vi "FormCalibra9.vi"() -> ()   [LabVIEW 2014]
uses:
  testMachine.ctl
  mainMachine.ctl
  <vilib>/Analysis/baseanly.llb/Mean (DBL).vi
  <vilib>/express/express shared/transition.llb/Dynamic To Waveform Array.vi
  <vilib>/express/express signal manip/GetorSetDDTAttributes/Set DDT Attributes/SetT0.vi
  <vilib>/express/express shared/transition.llb/Waveform Array To Dynamic.vi
  <vilib>/measure/mamon.llb/Trigger Detection for 1 Channel.vi
  <vilib>/express/express signal manip/GetorSetDDTAttributes/Set DDT Attributes/Set DDT Properties.xnode
  <vilib>/Analysis/NI_AALBase.lvlib
  <resource>/objmgr/daqmx.rc
  <vilib>/measure/NI_MAPro.lvlib
panel:
  out "editDistance":dbl caption="Distancia (m)" format="%#_4f"
  in  "Lower level":dbl
  in  "hysteresis":dbl format="%.2p"
  in  "level":dbl format="%.2p"
  out "rpm":bool
  out "deviceName":tag
  out "editTotalWaitLimit":u8
  out "editCountWaitLimit":u8
  out "ledWaitState":bool caption="Wait State"
  out "sliderWaitUpperTime":u8(slide) max=50 scale=0.0..100.0
  out "slideWaitLowerTime":u8(slide) max=30 scale=0.0..100.0
  out "slideWaitTime":u8(slide) scale=0.0..100.0
  out "labelTestTime":string caption="Tempo total de ensaio"
  in  "buttonAcquisition":bool
  in  "editSetWaitTime":u8 caption="Tempo entre ciclos (s)" step=1 format="%0d"
  in  "stop":bool
  out "error out":errorcluster
  out "ledAcquireState":bool caption="Acquire State"
  out "editTotalLowerLimit":u8
  out "editCountLowerLimit":u8
  out "editTotalUpperLimit":u8
  out "editCountUpperLimit":u8
  out "ledEnsaio 3":bool
  out "ledBrakeState":bool caption="Brake State"
  out "ledExitState":bool caption="Exit State"
  out "ledMotorState":bool caption="Motor State"
  out "ledInit2State":bool caption="Init State"
  out "ledBlockState":bool caption="Block State"
  out "ledRunningState":bool caption="Running State"
  out "ledReadyState":bool caption="Ready State"
  out "ledInitState":bool caption="Init State"
  out "mainMachine":T1
  out "testMachine":T2=enum."finish"
  in  "editSetPathToFile":path
  in  "buttonStop":bool
  in  "buttonStart":bool
  out "graphForce":dynamicdata(graph)
  in  "editOffsetForce":dbl caption="Tara" min=0.0 max=100.0 step=0.1
  in  "editSetForce":dbl caption="Fator de conversão"
  out "editForce":dbl caption="Força (Kgf)" format="%#_4f"
  out "graphSpeed":dynamicdata(graph)
  in  "editSetSpeed":dbl caption="Fator de conversão"
  out "editSpeed":dbl caption="Velocidade (km/h)" format="%#_4f"
  out "editEngineSpeed":dbl caption="Rotação (RPM)" format="%#_4f"
  in  "buttonMotor":bool
  in  "buttonBrake":bool
  in  "editSetWaitLowerTime":u8 caption="Tempo de espera (s)"
  in  "editSetWaitUpperTime":u8=3 caption="Tempo de espera (s)"
  in  "editSetNumberOfCycles":u16 caption="Número de ciclos" max=999 step=1 format="%0d"
  in  "editSetLowerLimit":u32 caption="Limite inferior (km/h)"
  in  "editSetUpperLimit":u32 caption="Limite superior (km/h)"
  out "editTempB":dbl caption="Temperatura B (ºC)"
  out "editTempA":dbl caption="Temperatura A (ºC)"
  in  "editSetTempRef":dbl caption="Offset referência" step=0.01 format="%#_2f"
  out "editTempRef":dbl caption="Referência (ºC)"
  out "ledMotor":bool
  out "ledBrake":bool
  out "ledEnsaio":bool
  out "labelTotalCycle":string
  out "labelCurrentCycle":string
  out "labelSystemTitle":string
  in  "editCurrCycleCtr":u32
  in  "velocidade 2":u32
  out "velocidade":u32
  # "Bancada de Frenagem - Ensaio"
  # "Ensaio"
  # "Temperatura"
  # "Rotação"
  # "Célula de Carga"
  # "Configurações do ensaio"
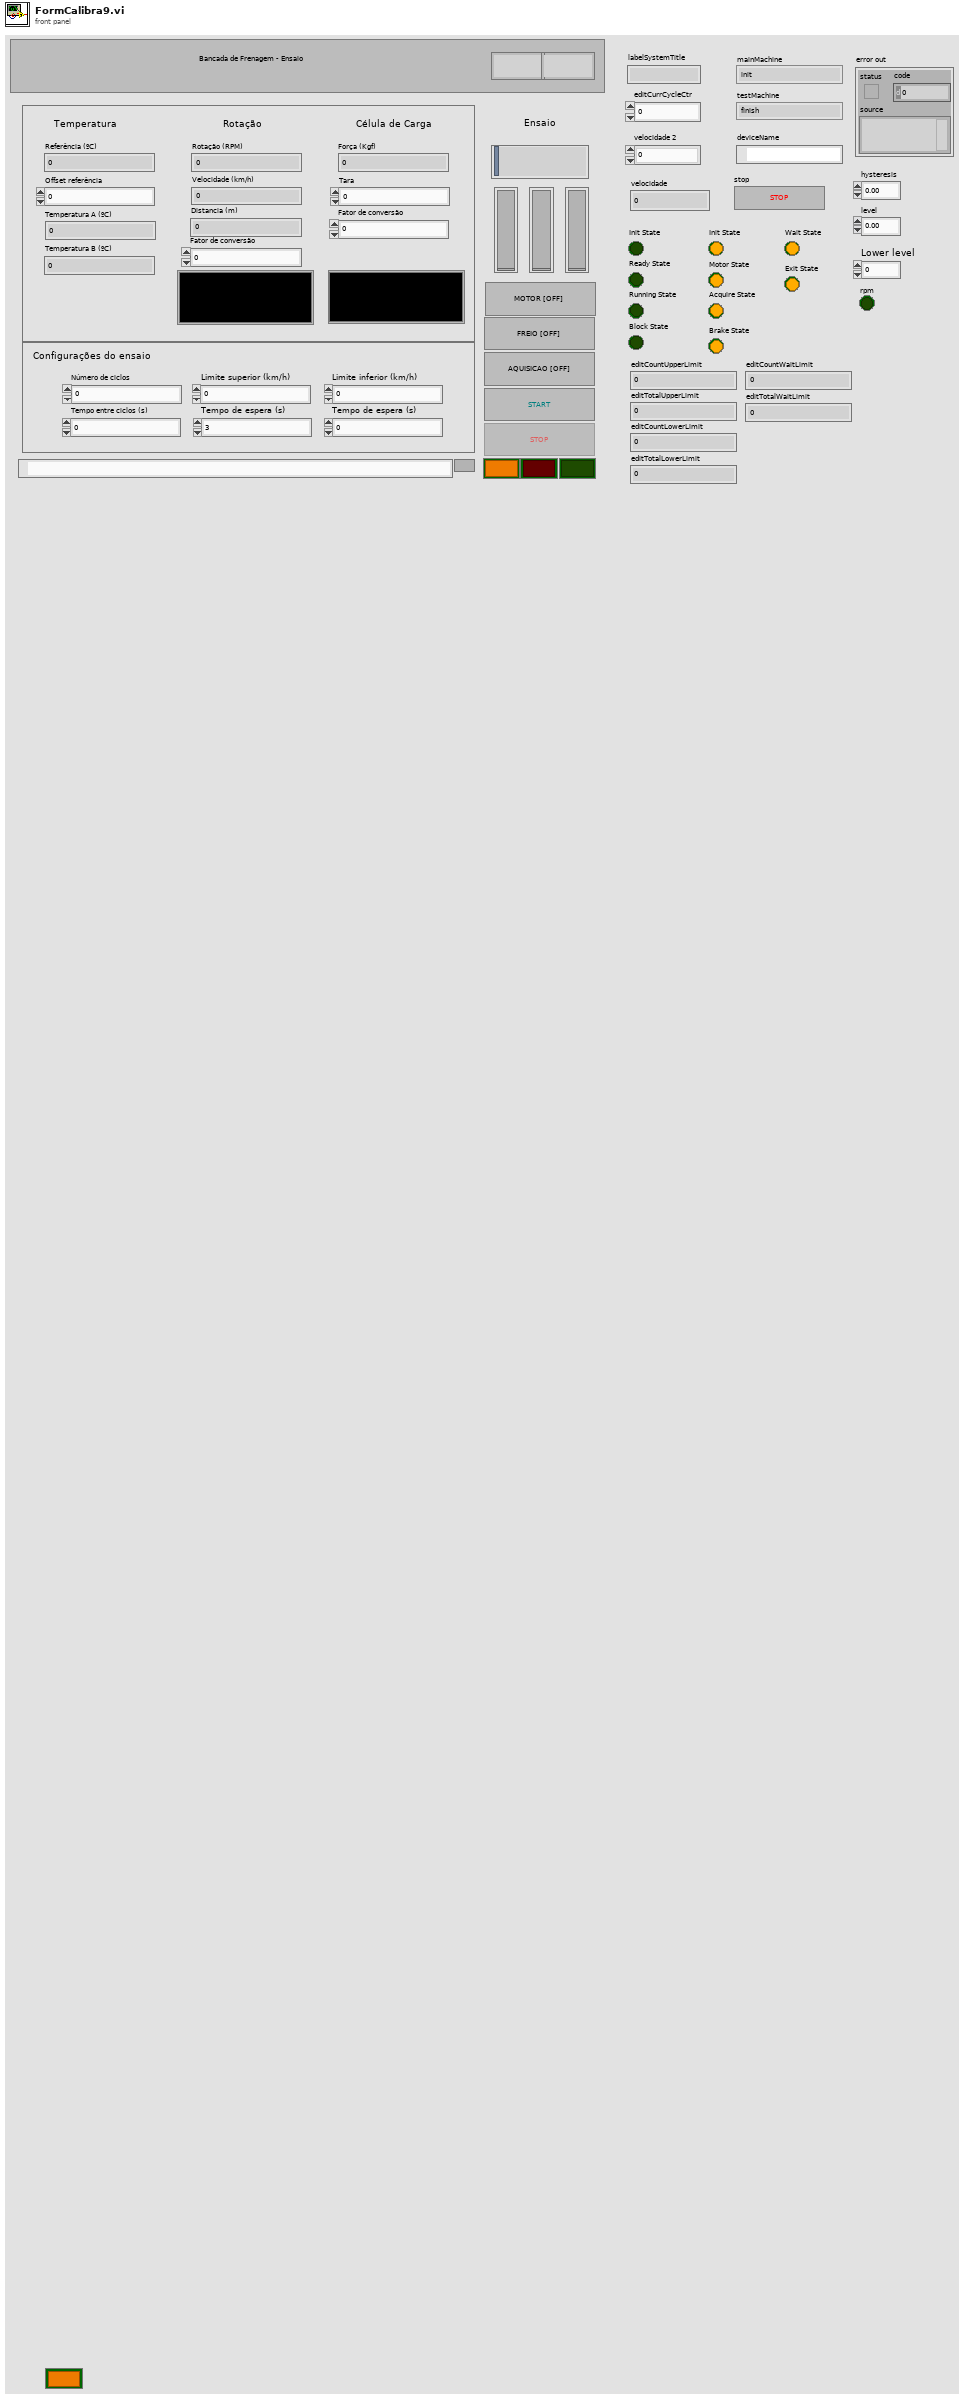
[diagram p1: front panel]
types:
  T1 = typedef "mainMachine.ctl" = enum16{"init", "ready", "running", "blocked", "finish"}
  T2 = typedef "testMachine.ctl" = enum16{"init", "motor", "motor acquire", "brake", "brake acquire", "wait ", "finish", "exit"}
  T3 = enum8{"Enabled", "Disabled", "Disabled and Grayed Out"}
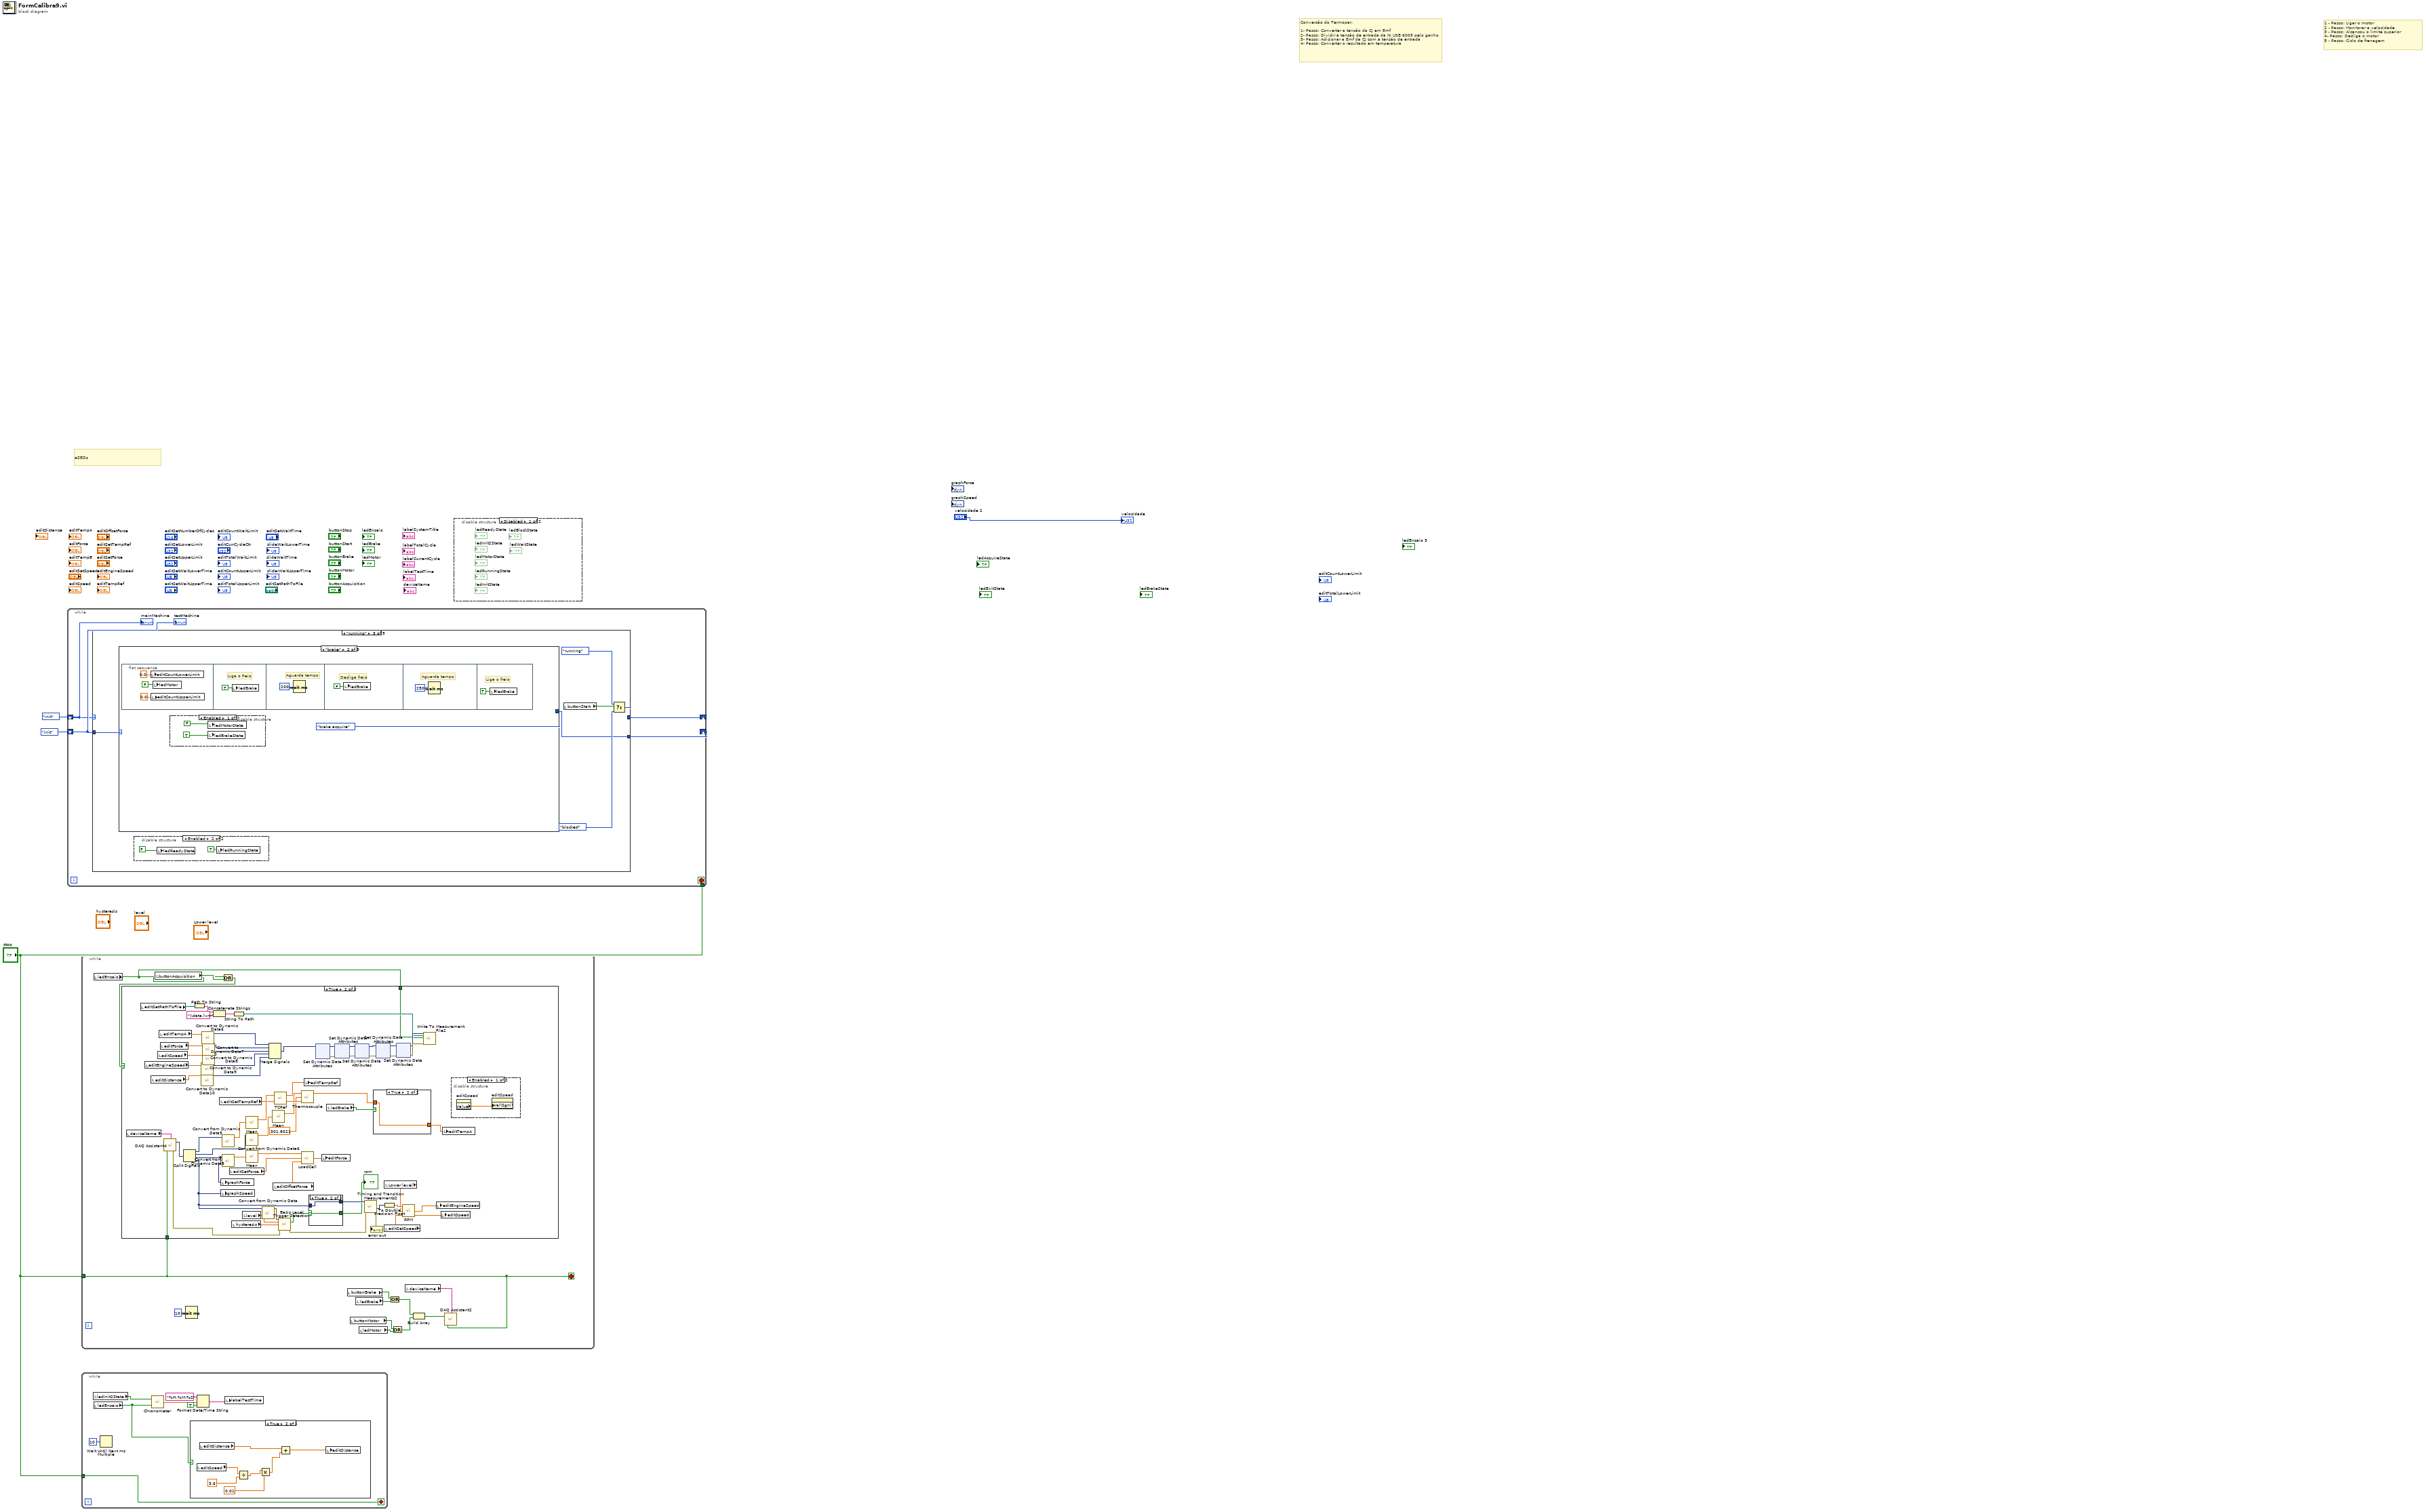
[diagram p0: block diagram]
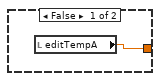
[diagram p5: hidden frame]
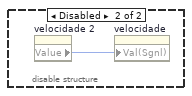
[diagram p7: hidden frame]
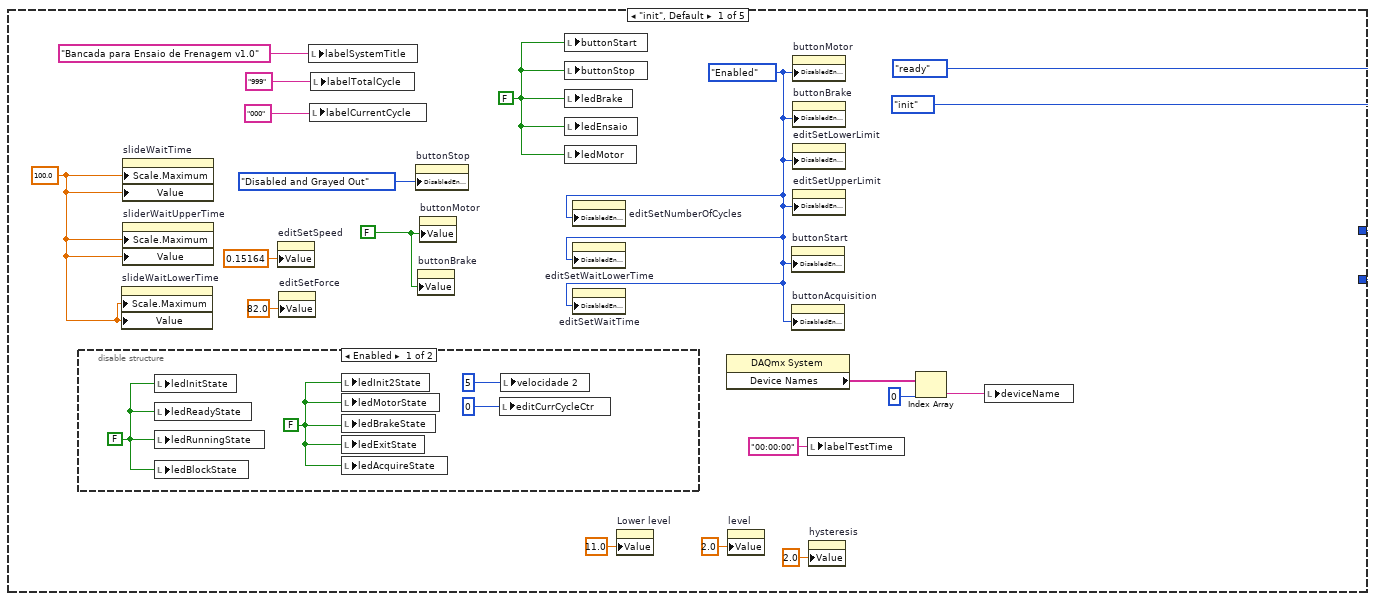
[diagram p8: hidden frame]
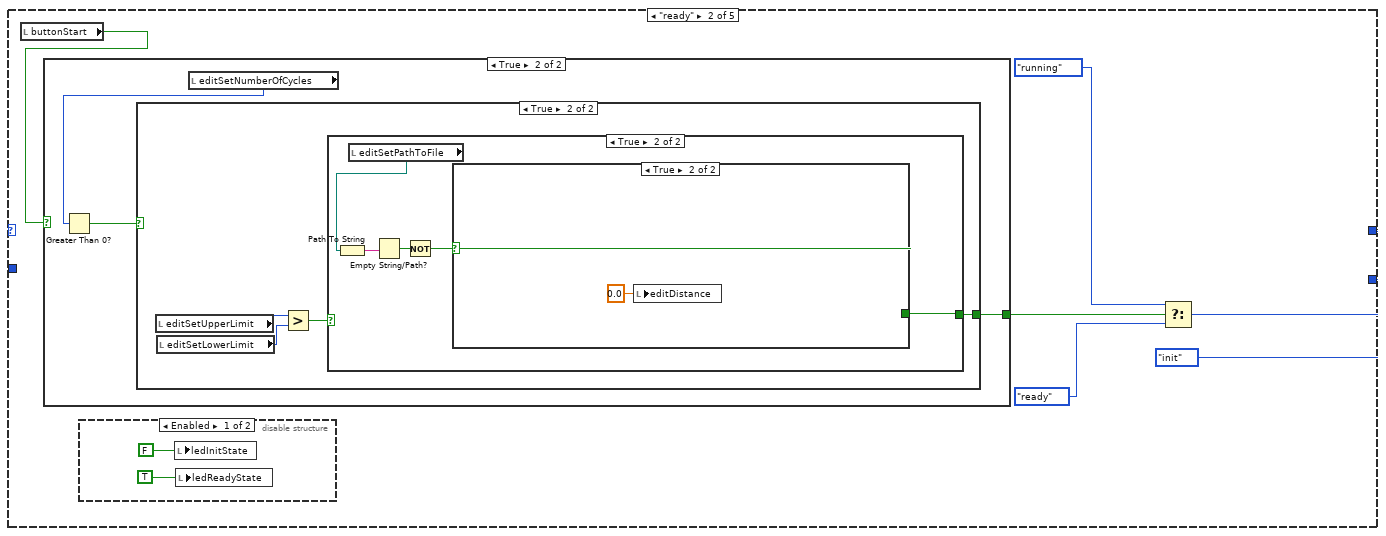
[diagram p10: hidden frame]
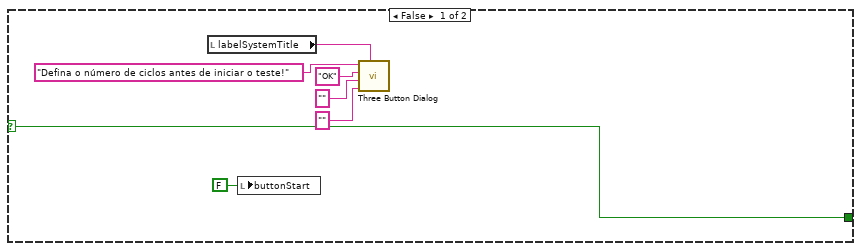
[diagram p13: hidden frame]
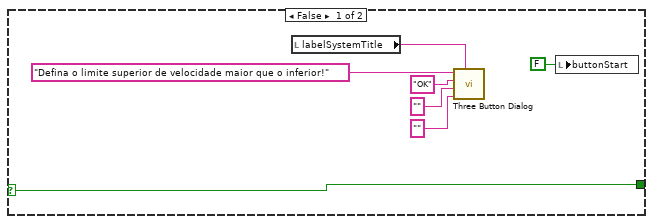
[diagram p14: hidden frame]
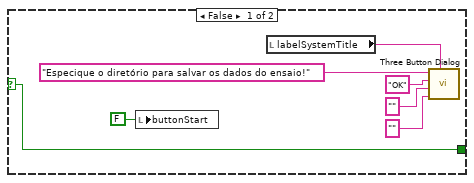
[diagram p15: hidden frame]
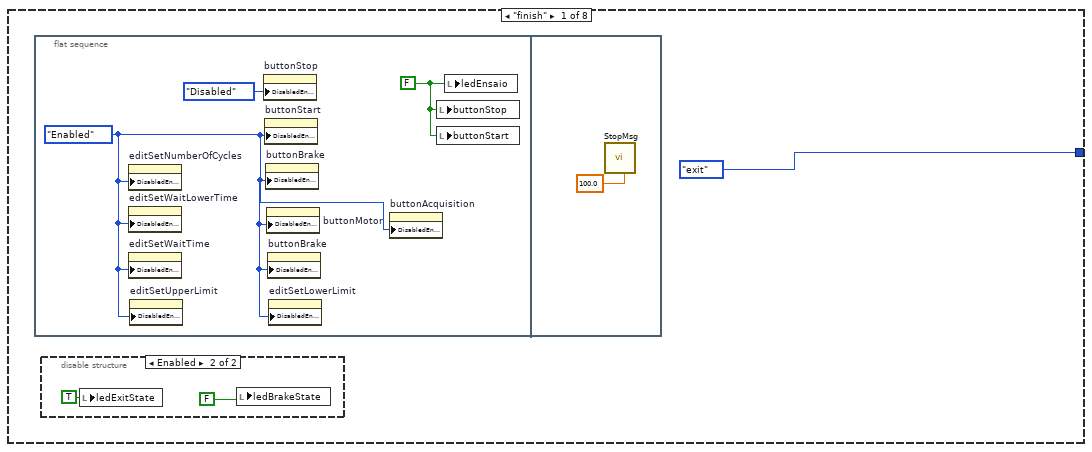
[diagram p17: hidden frame]
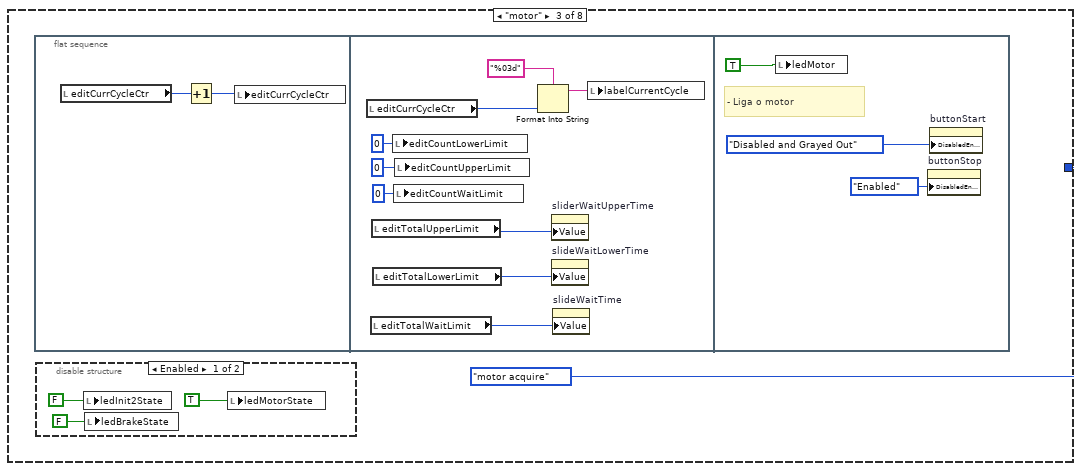
[diagram p20: hidden frame]
diagram:
  # "eSEDs"
  # "1 - Passo: Ligar o motor\n2 - Passo: Monitorar a velocidade\n3 - Passo: Alcancou o limite superior\n4- Passo: Desliga o motor\n5 - Passo: Ciclo de frenagem"
  # "Conversão do Termopar:\n\n1- Passo: Converter a tensão da CJ em Emf\n2- Passo: Dividir a tensão de entrada da NI USB 6009 pelo ganho\n3- Passo: Adicionar a Emf da CJ com a tensão de entrada\n4- Passo: Converter o resultado em temperatura"
  n1 = while {
    shift-right: [w9] -> _
    shift-left: mainMachine."init" ("mainMachine") -> [w6]
    shift-right: [w8] -> _
    shift-left: testMachine."init" ("testMachine") -> [w7]
    tunnel: "stop" -> [w5]
    stop <- w5 stop-if-true
    n2 = case shown="\"running\"" w6 {
      tunnel: [mainMachine."ready" ("mainMachine") w33 w79 w223 mainMachine."finish" ("mainMachine")] -> w9
      tunnel: [testMachine."init" ("testMachine") testMachine."init" ("testMachine") w78 testMachine."init" ("testMachine") testMachine."init" ("testMachine")] -> w8
      tunnel: w7 -> [_ _ w77 _ _]
      frame "init", Default {
        w19 = 100.0 ("Scale.Range:Maximum")
        w20 = T3."Enabled" ("Disabled")
        w21 = FALSE ("buttonMotor")
        w27 = FALSE ("motor")
        n3 = disable-structure shown="Enabled" {
          frame Enabled {
            w29 = FALSE
            w30 = FALSE
            n4 = local write "ledInitState"(w30) -> ()
            n5 = local write "ledReadyState"(w30) -> ()
            n6 = local write "ledRunningState"(w30) -> ()
            n7 = local write "ledBlockState"(w30) -> ()
            n8 = local write "ledInit2State"(w29) -> ()
            n9 = local write "ledMotorState"(w29) -> ()
            n10 = local write "ledBrakeState"(w29) -> ()
            n11 = local write "ledExitState"(w29) -> ()
            n12 = local write "ledAcquireState"(w29) -> ()
            n13 = local write "editCurrCycleCtr"(u32 0 ("currentCycleCtr")) -> ()
            n14 = local write "velocidade 2"(u32 5 ("velocidade 2")) -> ()
          }
          frame Disabled {
          }
        }
        n15 = property on="slideWaitLowerTime" class="Slide (strict)"("Scale.Maximum"=w19, "Value"=w19) -> ()  [unwired: 2 in, 2 out]
        n16 = property on="slideWaitTime" class="Slide (strict)"("Scale.Maximum"=w19, "Value"=w19) -> ()  [unwired: 2 in, 2 out]
        n17 = property on="sliderWaitUpperTime" class="Slide (strict)"("Scale.Maximum"=w19, "Value"=w19) -> ()  [unwired: 2 in, 2 out]
        n18 = property on="editSetSpeed" class="DigNum (strict)"("Value"=0.15164 ("editSetSpeed")) -> ()  [unwired: 2 in, 2 out]
        n19 = property on="editSetForce" class="DigNum (strict)"("Value"=82.0 ("editSetForce")) -> ()  [unwired: 2 in, 2 out]
        n20 = local write "labelSystemTitle"("Bancada para Ensaio de Frenagem v1.0" ("systemTitle")) -> ()
        n21 = local write "labelCurrentCycle"("000" ("currentCycle")) -> ()
        n22 = local write "labelTotalCycle"("999" ("totalCycle")) -> ()
        n23 = property on="buttonStop" class="Bool (strict)"("DisabledEnum"=T3."Disabled and Grayed Out" ("Disabled")) -> ()  [unwired: 2 in, 2 out]
        n24 = property on="buttonBrake" class="Bool (strict)"("Value"=w21) -> ()  [unwired: 2 in, 2 out]
        n25 = property on="buttonMotor" class="Bool (strict)"("Value"=w21) -> ()  [unwired: 2 in, 2 out]
        n26 = local write "buttonStart"(w27) -> ()
        n27 = local write "buttonStop"(w27) -> ()
        n28 = local write "ledBrake"(w27) -> ()
        n29 = local write "ledEnsaio"(w27) -> ()
        n30 = local write "ledMotor"(w27) -> ()
        n31 = property on="editSetNumberOfCycles" class="DigNum (strict)"("DisabledEnum"=w20) -> ()  [unwired: 2 in, 2 out]
        n32 = property on="editSetWaitLowerTime" class="DigNum (strict)"("DisabledEnum"=w20) -> ()  [unwired: 2 in, 2 out]
        n33 = property on="editSetWaitTime" class="DigNum (strict)"("DisabledEnum"=w20) -> ()  [unwired: 2 in, 2 out]
        n34 = property on="Lower level" class="DigNum (strict)"("Value"=11.0 ("Lower level")) -> ()  [unwired: 2 in, 2 out]
        n35 = property class="DAQmx System"() -> ("Device Names"=w18:tag[])  [unwired: 2 in, 2 out]
        n36 = property on="level" class="DigNum (strict)"("Value"=2.0 ("level")) -> ()  [unwired: 2 in, 2 out]
        n37 = property on="buttonStart" class="Bool (strict)"("DisabledEnum"=w20) -> ()  [unwired: 2 in, 2 out]
        n38 = property on="buttonAcquisition" class="Bool (strict)"("DisabledEnum"=w20) -> ()  [unwired: 2 in, 2 out]
        n39 = property on="buttonMotor" class="Bool (strict)"("DisabledEnum"=w20) -> ()  [unwired: 2 in, 2 out]
        n40 = property on="buttonBrake" class="Bool (strict)"("DisabledEnum"=w20) -> ()  [unwired: 2 in, 2 out]
        n41 = property on="editSetLowerLimit" class="DigNum (strict)"("DisabledEnum"=w20) -> ()  [unwired: 2 in, 2 out]
        n42 = property on="editSetUpperLimit" class="DigNum (strict)"("DisabledEnum"=w20) -> ()  [unwired: 2 in, 2 out]
        n43 = local write "labelTestTime"("00:00:00" ("labelTestTime")) -> ()
        n44 = property on="hysteresis" class="DigNum (strict)"("Value"=2.0 ("hysteresis")) -> ()  [unwired: 2 in, 2 out]
        n45 = Index Array(array=w18, index=0) -> (element=w16:tag)
        n46 = local write "deviceName"(w16) -> ()
      }
      frame "ready" {
        n47 = local read "buttonStart"() -> (w36:bool)
        n48 = case shown="True" w36 {
          selector: w36 -> [w41 _]
          tunnel: [w41 w42] -> w35
          frame False {
          }
          frame True {
            n49 = local read "editSetNumberOfCycles"() -> (w43:u16)
            n50 = Greater Than 0?(x=w43) -> (x > 0?=w44:bool)
            n51 = case shown="True" w44 {
              selector: w44 -> [w51 _]
              tunnel: [w51 w52] -> w42
              frame False {
                n52 = local read "labelSystemTitle"() -> (w46:string)
                n53 = local write "buttonStart"(FALSE ("startButton")) -> ()
                n54 = call <vilib>:"Three Button Dialog.vi"("Window Title (\"\")"=w46, "Right Button Text (\"Cancel\")"="" ("Right Button Text (\"Cancel\")"), "Center Button Text (\"No\")"="" ("Center Button Text (\"No\")"), "Left Button Text (\"Yes\")"="OK" ("Left Button Text (\"Yes\")"), "message"="Defina o número de ciclos antes de iniciar o teste!") -> ()  [unwired: 6 in, 1 out]
              }
              frame True {
                n55 = local read "editSetUpperLimit"() -> (w54:u32)
                n56 = local read "editSetLowerLimit"() -> (w53:u32)
                n57 = Greater?(x=w54, y=w53) -> (0:w55:bool)
                n58 = case shown="True" w55 {
                  selector: w55 -> [w62 _]
                  tunnel: [w62 w65] -> w52
                  frame False {
                    n59 = local read "labelSystemTitle"() -> (w57:string)
                    n60 = call <vilib>:"Three Button Dialog.vi"("Window Title (\"\")"=w57, "Right Button Text (\"Cancel\")"="" ("Right Button Text (\"Cancel\")"), "Center Button Text (\"No\")"="" ("Center Button Text (\"No\")"), "Left Button Text (\"Yes\")"="OK" ("Left Button Text (\"Yes\")"), "message"="Defina o limite superior de velocidade maior que o inferior!") -> ()  [unwired: 6 in, 1 out]
                    n61 = local write "buttonStart"(FALSE ("startButton")) -> ()
                  }
                  frame True {
                    n62 = local read "editSetPathToFile"() -> (w67:path)
                    n63 = Path To String(path=w67) -> (string=w66:string)
                    n64 = Empty String/Path?(string/path=w66) -> (empty?=w64:bool)
                    n65 = Not(x=w64) -> (.not. x?=w63:bool)
                    n66 = case shown="True" w63 {
                      selector: w63 -> [w74 w76]
                      tunnel: [w74 w76] -> w65
                      frame False {
                        n67 = local write "buttonStart"(FALSE ("startButton")) -> ()
                        n68 = local read "labelSystemTitle"() -> (w69:string)
                        n69 = call <vilib>:"Three Button Dialog.vi"("Window Title (\"\")"=w69, "Right Button Text (\"Cancel\")"="" ("Right Button Text (\"Cancel\")"), "Center Button Text (\"No\")"="" ("Center Button Text (\"No\")"), "Left Button Text (\"Yes\")"="OK" ("Left Button Text (\"Yes\")"), "message"="Especique o diretório para salvar os dados do ensaio!") -> ()  [unwired: 6 in, 1 out]
                      }
                      frame True {
                        n70 = local write "editDistance"(0.0 ("editDistance")) -> ()
                      }
                    }
                  }
                }
              }
            }
          }
        }
        n71 = disable-structure shown="Enabled" {
          frame Enabled {
            n72 = local write "ledInitState"(FALSE ("ledReady")) -> ()
            n73 = local write "ledReadyState"(TRUE ("ledReady")) -> ()
          }
          frame Disabled {
          }
        }
        n74 = Select(t=mainMachine."running" ("mainMachine"), s=w35, f=mainMachine."ready" ("mainMachine")) -> (s? t:f=w33:T1)
      }
      frame "running" {
        n75 = case shown="\"brake\"" w77 {
          tunnel: [testMachine."exit" ("testMachine") testMachine."brake acquire" ("testMachine") testMachine."motor acquire" ("testMachine") testMachine."motor" ("testMachine") w153 w173 testMachine."exit" ("testMachine") w206] -> w78
          frame "finish" {
            n76 = flat-sequence {
              frame #0 {
                w89 = FALSE ("ledReady")
                w88 = T3."Enabled" ("Disabled")
                n77 = property on="editSetNumberOfCycles" class="DigNum (strict)"("DisabledEnum"=w88) -> ()  [unwired: 2 in, 2 out]
                n78 = property on="editSetWaitLowerTime" class="DigNum (strict)"("DisabledEnum"=w88) -> ()  [unwired: 2 in, 2 out]
                n79 = property on="editSetWaitTime" class="DigNum (strict)"("DisabledEnum"=w88) -> ()  [unwired: 2 in, 2 out]
                n80 = property on="editSetUpperLimit" class="DigNum (strict)"("DisabledEnum"=w88) -> ()  [unwired: 2 in, 2 out]
                n81 = property on="buttonStop" class="Bool (strict)"("DisabledEnum"=T3."Disabled" ("Disabled")) -> ()  [unwired: 2 in, 2 out]
                n82 = property on="buttonStart" class="Bool (strict)"("DisabledEnum"=w88) -> ()  [unwired: 2 in, 2 out]
                n83 = property on="buttonBrake" class="Bool (strict)"("DisabledEnum"=w88) -> ()  [unwired: 2 in, 2 out]
                n84 = property on="buttonMotor" class="Bool (strict)"("DisabledEnum"=w88) -> ()  [unwired: 2 in, 2 out]
                n85 = property on="buttonBrake" class="Bool (strict)"("DisabledEnum"=w88) -> ()  [unwired: 2 in, 2 out]
                n86 = property on="editSetLowerLimit" class="DigNum (strict)"("DisabledEnum"=w88) -> ()  [unwired: 2 in, 2 out]
                n87 = property on="buttonAcquisition" class="Bool (strict)"("DisabledEnum"=w88) -> ()  [unwired: 2 in, 2 out]
                n88 = local write "buttonStop"(w89) -> ()
                n89 = local write "buttonStart"(w89) -> ()
                n90 = local write "ledEnsaio"(w89) -> ()
              }
              frame #1 {
                n91 = call "StopMsg.vi"("Max Value (100)"=100.0) -> ()  [unwired: 8 in, 2 out]
              }
            }
            n92 = disable-structure shown="Enabled" {
              frame Disabled {
              }
              frame Enabled {
                n93 = local write "ledExitState"(TRUE ("ledReady")) -> ()
                n94 = local write "ledBrakeState"(FALSE ("ledReady")) -> ()
              }
            }
          }
          frame "brake" {
            n95 = flat-sequence {
              frame #0 {
                n96 = local write "editCountLowerLimit"(0.0 ("editCountUpperLimit")) -> ()
                n97 = local write "editCountUpperLimit"(0.0 ("editCountUpperLimit")) -> ()
                n98 = local write "ledMotor"(FALSE ("motor")) -> ()
              }
              frame #1 {
                # "Liga o freio"
                n99 = local write "ledBrake"(TRUE ("freio")) -> ()
              }
              frame #2 {
                # "Aguarda tempo"
                n100 = Wait (ms)(milliseconds to wait=u32 200) -> ()  [unwired: 1 out]
              }
              frame #3 {
                # "Desliga freio"
                n101 = local write "ledBrake"(FALSE ("freio")) -> ()
              }
              frame #4 {
                # "Aguarda tempo"
                n102 = Wait (ms)(milliseconds to wait=u32 250) -> ()  [unwired: 1 out]
              }
              frame #5 {
                # "Liga o freio"
                n103 = local write "ledBrake"(TRUE ("freio")) -> ()
              }
            }
            n104 = disable-structure shown="Enabled" {
              frame Enabled {
                n105 = local write "ledMotorState"(FALSE ("ledReady")) -> ()
                n106 = local write "ledBrakeState"(TRUE ("ledReady")) -> ()
              }
              frame Disabled {
              }
            }
          }
          frame "motor" {
            n107 = flat-sequence {
              frame #0 {
                n108 = local read "editCurrCycleCtr"() -> (w108:u32)
                n109 = Increment(x=w108) -> (x+1=w107:u32)
                n110 = local write "editCurrCycleCtr"(w107) -> ()
              }
              frame #1 {
                n111 = local read "editCurrCycleCtr"() -> (w115:u32)
                n112 = local read "editTotalWaitLimit"() -> (w109:u8)
                n113 = local read "editTotalUpperLimit"() -> (w111:u8)
                n114 = local read "editTotalLowerLimit"() -> (w110:u8)
                n115 = local write "editCountLowerLimit"(u8 0 ("editCountLowerLimit")) -> ()
                n116 = local write "editCountWaitLimit"(u8 0 ("editCountWaitLimit")) -> ()
                n117 = local write "editCountUpperLimit"(u8 0 ("editCountUpperLimit")) -> ()
                n118 = Format Into String(format string="%03d", w115) -> (resulting string=w116:string)  [unwired: 2 in, 1 out]
                n119 = property on="sliderWaitUpperTime" class="Slide (strict)"("Value"=w111) -> ()  [unwired: 2 in, 2 out]
                n120 = property on="slideWaitLowerTime" class="Slide (strict)"("Value"=w110) -> ()  [unwired: 2 in, 2 out]
                n121 = property on="slideWaitTime" class="Slide (strict)"("Value"=w109) -> ()  [unwired: 2 in, 2 out]
                n122 = local write "labelCurrentCycle"(w116) -> ()
              }
              frame #2 {
                # "- Liga o motor"
                n123 = local write "ledMotor"(TRUE ("motor")) -> ()
                n124 = property on="buttonStop" class="Bool (strict)"("DisabledEnum"=T3."Enabled" ("Disabled")) -> ()  [unwired: 2 in, 2 out]
                n125 = property on="buttonStart" class="Bool (strict)"("DisabledEnum"=T3."Disabled and Grayed Out" ("Disabled")) -> ()  [unwired: 2 in, 2 out]
              }
            }
            n126 = disable-structure shown="Enabled" {
              frame Enabled {
                n127 = local write "ledInit2State"(FALSE ("ledReady")) -> ()
                n128 = local write "ledBrakeState"(FALSE ("ledReady")) -> ()
                n129 = local write "ledMotorState"(TRUE ("ledReady")) -> ()
              }
              frame Disabled {
              }
            }
          }
          frame "init", Default {
            n130 = stacked-sequence {
              frame #0 {
                w128 = FALSE ("ensaio")
                n131 = property on="buttonBrake" class="Bool (strict)"("Value"=w128) -> ()  [unwired: 2 in, 2 out]
                n132 = local write "ledMotor"(w128) -> ()
                n133 = local write "ledBrake"(w128) -> ()
                n134 = property on="buttonMotor" class="Bool (strict)"("Value"=w128) -> ()  [unwired: 2 in, 2 out]
                n135 = local read "editSetNumberOfCycles"() -> (w135:u16)
                n136 = local read "editSetWaitLowerTime"() -> (w129:u8)
                n137 = local read "editSetWaitUpperTime"() -> (w132:u8)
                n138 = local read "editSetWaitTime"() -> (w123:u8)
                n139 = Multiply(x=w123, y=u32 10) -> (x*y=w124:u32)
                n140 = Multiply(x=w129, y=u32 10) -> (x*y=w127:u32)
                n141 = Format Into String(format string="%03d", w135) -> (resulting string=w136:string)  [unwired: 2 in, 1 out]
                n142 = Multiply(x=w132, y=u32 10) -> (x*y=w126:u32)
                n143 = local write "editTotalLowerLimit"(w127) -> ()
                n144 = local write "editTotalUpperLimit"(w126) -> ()
                n145 = local write "editTotalWaitLimit"(w124) -> ()
                n146 = local write "labelTotalCycle"(w136) -> ()
                n147 = local write "editCurrCycleCtr"(u32 0 ("currentCycleCtr")) -> ()
                n148 = local write "labelCurrentCycle"("000" ("currentCycle")) -> ()
              }
              frame #1 {
                w144 = T3."Disabled" ("Disabled")
                n149 = property on="editSetNumberOfCycles" class="DigNum (strict)"("DisabledEnum"=w144) -> ()  [unwired: 2 in, 2 out]
                n150 = property on="editSetWaitLowerTime" class="DigNum (strict)"("DisabledEnum"=w144) -> ()  [unwired: 2 in, 2 out]
                n151 = property on="editSetWaitTime" class="DigNum (strict)"("DisabledEnum"=w144) -> ()  [unwired: 2 in, 2 out]
                n152 = local read "editTotalUpperLimit"() -> (w147:u8)
                n153 = property on="sliderWaitUpperTime" class="Slide (strict)"("Scale.Maximum"=w147, "Scale.Minimum"=0.0 ("Scale.Range:Minimum"), "Scale.Increment"=1.0 ("Scale.Range:Increment"), "Value"=w147) -> ()  [unwired: 2 in, 2 out]
                n154 = property on="buttonAcquisition" class="Bool (strict)"("DisabledEnum"=w144) -> ()  [unwired: 2 in, 2 out]
                n155 = local read "editTotalLowerLimit"() -> (w141:u8)
                n156 = property on="slideWaitLowerTime" class="Slide (strict)"("Scale.Maximum"=w141, "Scale.Minimum"=0.0 ("Scale.Range:Minimum"), "Scale.Increment"=1.0 ("Scale.Range:Increment"), "Value"=w141) -> ()  [unwired: 2 in, 2 out]
                n157 = local read "editTotalWaitLimit"() -> (w138:u8)
                n158 = property on="slideWaitTime" class="Slide (strict)"("Scale.Maximum"=w138, "Scale.Minimum"=0.0 ("Scale.Range:Minimum"), "Scale.Increment"=1.0 ("Scale.Range:Increment"), "Value"=w138) -> ()  [unwired: 2 in, 2 out]
                n159 = call "StarMsg.vi"("Show"=TRUE, "Max Value (100)"=100.0) -> ()  [unwired: 7 in, 2 out]
                n160 = property on="buttonMotor" class="Bool (strict)"("DisabledEnum"=w144) -> ()  [unwired: 2 in, 2 out]
                n161 = property on="buttonBrake" class="Bool (strict)"("DisabledEnum"=w144) -> ()  [unwired: 2 in, 2 out]
                n162 = property on="editSetLowerLimit" class="DigNum (strict)"("DisabledEnum"=w144) -> ()  [unwired: 2 in, 2 out]
                n163 = property on="editSetUpperLimit" class="DigNum (strict)"("DisabledEnum"=w144) -> ()  [unwired: 2 in, 2 out]
              }
              frame #2 {
                n164 = local write "ledEnsaio"(TRUE ("ensaio")) -> ()
              }
            }
            n165 = disable-structure shown="Enabled" {
              frame Enabled {
                n166 = local write "ledInit2State"(TRUE ("ledReady")) -> ()
              }
              frame Disabled {
              }
            }
          }
          frame "motor acquire" {
            n167 = disable-structure shown="Enabled" {
              frame Enabled {
                n168 = local read "ledAcquireState"() -> (w162:bool)
                n169 = Not(x=w162) -> (.not. x?=w161:bool)
                n170 = local write "ledAcquireState"(w161) -> ()
              }
              frame Disabled {
              }
            }
            n171 = Wait (ms)(milliseconds to wait=u32 100) -> ()  [unwired: 1 out]
            n172 = disable-structure shown="Enabled" {
              disable-tunnel: [w159 w160] -> w152
              frame Enabled {
                n173 = property on="editSpeed" class="DigNum (strict)"() -> ("Value"=w159:dbl)  [unwired: 2 in, 2 out]
              }
              frame Disabled {
                n174 = property on="velocidade" class="DigNum (strict)"() -> ("Value"=w160:u32)  [unwired: 2 in, 2 out]
              }
            }
            n175 = property on="editSetUpperLimit" class="DigNum (strict)"() -> ("Value"=w151:u32)  [unwired: 2 in, 2 out]
            n176 = Greater Or Equal?(x=w152, y=w151) -> (x >= y?=w157:bool)
            n177 = case shown="True" w157 {
              selector: w157 -> [w163 _]
              tunnel: [w163 w164] -> w156
              frame False {
              }
              frame True {
                n178 = flat-sequence {
                  tunnel: [w169] -> w164
                  frame #0 {
                    n179 = local read "editCountUpperLimit"() -> (w167:u8)
                    n180 = Increment(x=w167) -> (x+1=w165:u8)
                    n181 = local write "editCountUpperLimit"(w165) -> ()
                    n182 = local read "editTotalUpperLimit"() -> (w166:u8)
                    n183 = Subtract(x=w166, y=w165) -> (x-y=w168:u8)
                    n184 = property on="sliderWaitUpperTime" class="Slide (strict)"("Value"=w168) -> ()  [unwired: 2 in, 2 out]
                  }
                  frame #1 {
                    n185 = local read "editCountUpperLimit"() -> (w171:u8)
                    n186 = local read "editTotalUpperLimit"() -> (w170:u8)
                    n187 = Greater Or Equal?(x=w171, y=w170) -> (x >= y?=w169:bool)
                  }
                }
              }
            }
            n188 = Select(t=testMachine."brake" ("testMachine"), s=w156, f=testMachine."motor acquire" ("testMachine")) -> (s? t:f=w153:T2)
          }
          frame "brake acquire" {
            n189 = disable-structure shown="Enabled" {
              frame Enabled {
                n190 = local read "ledAcquireState"() -> (w181:bool)
                n191 = Not(x=w181) -> (.not. x?=w180:bool)
                n192 = local write "ledAcquireState"(w180) -> ()
              }
              frame Disabled {
              }
            }
            n193 = Wait (ms)(milliseconds to wait=u32 100) -> ()  [unwired: 1 out]
            n194 = disable-structure shown="Enabled" {
              disable-tunnel: [w182 w183] -> w172
              frame Enabled {
                n195 = property on="editSpeed" class="DigNum (strict)"() -> ("Value"=w182:dbl)  [unwired: 2 in, 2 out]
              }
              frame Disabled {
                n196 = property on="velocidade" class="DigNum (strict)"() -> ("Value"=w183:u32)  [unwired: 2 in, 2 out]
              }
            }
            n197 = property on="editSetLowerLimit" class="DigNum (strict)"() -> ("Value"=w174:u32)  [unwired: 2 in, 2 out]
            n198 = Less Or Equal?(x=w172, y=w174) -> (x <= y?=w178:bool)
            n199 = case shown="True" w178 {
              selector: w178 -> [w184 _]
              tunnel: [w184 w185] -> w176
              frame False {
              }
              frame True {
                n200 = flat-sequence {
                  tunnel: [w191] -> w186
                  tunnel: w186 -> [w195]
                  tunnel: [w194] -> w185
                  frame #0 {
                    n201 = local read "editCountLowerLimit"() -> (w190:u8)
                    n202 = Increment(x=w190) -> (x+1=w189:u8)
                    n203 = local write "editCountLowerLimit"(w189) -> ()
                    n204 = local read "editTotalLowerLimit"() -> (w188:u8)
                    n205 = Subtract(x=w188, y=w189) -> (x-y=w187:u8)
                    n206 = property on="slideWaitLowerTime" class="Slide (strict)"("Value"=w187) -> ()  [unwired: 2 in, 2 out]
                  }
                  frame #1 {
                    n207 = local read "editCountLowerLimit"() -> (w193:u8)
                    n208 = local read "editTotalLowerLimit"() -> (w192:u8)
                    n209 = Greater Or Equal?(x=w193, y=w192) -> (x >= y?=w191:bool)
                  }
                  frame #2 {
                    n210 = case shown="True" w195 {
                      selector: w195 -> [w196 w197]
                      tunnel: [w196 w197] -> w194
                      frame False {
                      }
                      frame True {
                        # "- Desliga o freio"
                        n211 = local write "ledBrake"(FALSE ("freio")) -> ()
                      }
                    }
                  }
                }
              }
            }
            n212 = Select(t=testMachine."wait " ("testMachine"), s=w176, f=testMachine."brake acquire" ("testMachine")) -> (s? t:f=w173:T2)
          }
          frame "exit" {
          }
          frame "wait " {
            # "- Aguarda 0.5s \n- Atualiza o numero de ciclos"
            n213 = flat-sequence {
              tunnel: [w212] -> w200
              frame #0 {
                n214 = local read "editCountWaitLimit"() -> (w208:u8)
                n215 = Increment(x=w208) -> (x+1=w209:u8)
                n216 = local write "editCountWaitLimit"(w209) -> ()
                n217 = local read "editTotalWaitLimit"() -> (w211:u8)
                n218 = Subtract(x=w211, y=w209) -> (x-y=w210:u8)
                n219 = property on="slideWaitTime" class="Slide (strict)"("Value"=w210) -> ()  [unwired: 2 in, 2 out]
              }
              frame #1 {
                n220 = local read "editCountWaitLimit"() -> (w214:u8)
                n221 = local read "editTotalWaitLimit"() -> (w213:u8)
                n222 = Greater Or Equal?(x=w214, y=w213) -> (x >= y?=w212:bool)
              }
            }
            n223 = disable-structure shown="Enabled" {
              frame Enabled {
                n224 = local read "ledWaitState"() -> (w221:bool)
                n225 = Not(x=w221) -> (.not. x?=w220:bool)
                n226 = local write "ledBrakeState"(FALSE ("ledBrakeState")) -> ()
                n227 = local write "ledWaitState"(w220) -> ()
              }
              frame Disabled {
              }
            }
            n228 = Wait (ms)(milliseconds to wait=u32 100) -> ()  [unwired: 1 out]
            n229 = case shown="True" w200 {
              selector: w200 -> [w215 _]
              tunnel: [w215 w219] -> w201
              frame False {
              }
              frame True {
                n230 = local read "editSetNumberOfCycles"() -> (w217:u16)
                n231 = local read "editCurrCycleCtr"() -> (w216:u32)
                n232 = Greater Or Equal?(x=w216, y=w217) -> (x >= y?=w219:bool)
                n233 = Not(x=w219) -> (.not. x?=w218:bool)
                n234 = local write "ledEnsaio"(w218) -> ()
              }
            }
            n235 = Select(t=testMachine."motor" ("testMachine"), s=w200, f=testMachine."wait " ("testMachine")) -> (s? t:f=w202:T2)
            n236 = Select(t=testMachine."finish" ("testMachine"), s=w201, f=w202) -> (s? t:f=w206:T2)
          }
        }
        n237 = disable-structure shown="Enabled" {
          frame Disabled {
          }
          frame Enabled {
            n238 = local write "ledReadyState"(FALSE ("ledReady")) -> ()
            n239 = local write "ledRunningState"(TRUE ("ledReady")) -> ()
          }
        }
        n240 = local read "buttonStart"() -> (w82:bool)
        n241 = Select(t=mainMachine."running" ("mainMachine"), s=w82, f=mainMachine."blocked" ("mainMachine")) -> (s? t:f=w79:T1)
      }
      frame "blocked" {
        n242 = local read "buttonStart"() -> (w227:bool)
        n243 = Select(t=mainMachine."ready" ("mainMachine"), s=w227, f=mainMachine."blocked" ("mainMachine")) -> (s? t:f=w223:T1)
        n244 = local write "ledRunningState"(FALSE ("ledReady")) -> ()
        n245 = local write "ledBlockState"(TRUE ("ledReady")) -> ()
      }
      frame "finish" {
        n246 = local write "ledBlockState"(FALSE ("ledReady")) -> ()
      }
    }
    "mainMachine" <- w6
    "testMachine" <- w7
  }
  n247 = while {
    tunnel: "stop" -> [w240]
    stop <- w240 stop-if-true
    n248 = local read "ledInit2State"() -> (w235:bool)
    n249 = local read "ledEnsaio"() -> (w233:bool)
    n250 = Wait Until Next ms Multiple(millisecond multiple=u32 10) -> ()  [unwired: 1 out]
    n251 = call "Chronometer.vi"("start"=w233, "reset"=w235) -> ("Time"=w239:dbl)
    n252 = case shown="True" w233 {
      frame False {
      }
      frame True {
        n253 = local read "editSpeed"() -> (w245:dbl)
        n254 = local read "editDistance"() -> (w247:dbl)
        n255 = Divide(x=w245, y=3.6) -> (x/y=w243:dbl)
        n256 = Multiply(x=w243, y=0.01) -> (x*y=w242:dbl)
        n257 = Add(x=w247, y=w242) -> (x+y=w241:dbl)
        n258 = local write "editDistance"(w241) -> ()
      }
    }
    n259 = Format Date/Time String(time format string (%c)="%H:%M:%S", seconds (now)=w239, UTC format=TRUE) -> (date/time string=w236:string)
    n260 = local write "labelTestTime"(w236) -> ()
  }
  n261 = while {
    tunnel: "stop" -> [w253]
    stop <- w253 stop-if-true
    n262 = local read "ledEnsaio"() -> (w250:bool)
    n263 = local read "buttonAcquisition"() -> (w252:bool)
    n264 = Wait (ms)(milliseconds to wait=u32 10) -> ()  [unwired: 1 out]
    n265 = Or(x=w250, y=w252) -> (x .or. y?=w251:bool)
    n266 = case shown="True" w251 {
      tunnel: w253 -> [_ w285]
      tunnel: w250 -> [_ w284]
      frame False {
      }
      frame True {
        n267 = local read "deviceName"() -> (w283:tag)
        n268 = local read "editSetPathToFile"() -> (w305:path)
        n269 = local read "editEngineSpeed"() -> (w267:dbl)
        n270 = local read "editDistance"() -> (w268:dbl)
        n271 = local read "editSpeed"() -> (w265:dbl)
        n272 = local read "editTempA"() -> (w317:dbl)
        n273 = local read "editForce"() -> (w266:dbl)
        n274 = call "DAQ Assistant4"("stop (F)"=w285, "device name"=w283) -> ("data"=w287:dynamicdata, "error out"=w282:errorcluster)  [unwired: 14 in, 2 out]
        n275 = Split Signals(w287) -> (w264:dynamicdata, w263:dynamicdata, w262:dynamicdata, w261:dynamicdata)  [unwired: 4 in]
        n276 = Path To String(path=w305) -> (string=w304:string)
        n277 = call "Convert to Dynamic Data9"("Double"=w267) -> ("Dynamic Data Type"=w321:dynamicdata)  [unwired: 3 in]
        n278 = call "Convert to Dynamic Data10"("Double"=w268) -> ("Dynamic Data Type"=w322:dynamicdata)  [unwired: 3 in]
        n279 = call "Convert to Dynamic Data6"("Double"=w317) -> ("Dynamic Data Type"=w318:dynamicdata)  [unwired: 3 in]
        n280 = call "Convert to Dynamic Data7"("Double"=w266) -> ("Dynamic Data Type"=w319:dynamicdata)  [unwired: 3 in]
        n281 = call "Convert to Dynamic Data8"("Double"=w265) -> ("Dynamic Data Type"=w320:dynamicdata)  [unwired: 3 in]
        n282 = Concatenate Strings(w304, "\\data.lvm" ("string")) -> (w307:string)
        n283 = local read "editSetTempRef"() -> (w289:dbl)
        n284 = local write "graphForce"(w262) -> ()
        n285 = local write "graphSpeed"(w261) -> ()
        n286 = call "Convert from Dynamic Data5"("Dynamic Data Type"=w264) -> ("Array"=w302:dbl[])  [unwired: 3 in]
        n287 = call "Convert from Dynamic Data8"("Dynamic Data Type"=w262) -> ("Array"=w291:dbl[])  [unwired: 3 in]
        n288 = local read "editSetForce"() -> (w300:dbl)
        n289 = local read "hysteresis"() -> (w274:dbl)
        n290 = String To Path(string=w307) -> (path=w308:path)
        n291 = local read "level"() -> (w273:dbl)
        n292 = call-poly <vilib>:"Mean.vi"("X"=w302) -> ("mean"=w303:dbl)  [unwired: 1 out]
        n293 = call "Convert from Dynamic Data6"("Dynamic Data Type"=w263) -> ("Array"=w290:dbl[])  [unwired: 3 in]
        n294 = call-poly <vilib>:"Mean.vi"("X"=w291) -> ("mean"=w295:dbl)  [unwired: 1 out]
        n295 = call "Convert from Dynamic Data"("Dynamic Data Type"=w261) -> ("Waveform"=w279:waveform(dbl))  [unwired: 3 in]
        n296 = Merge Signals(w318, w319, w320, w321, w322) -> (w323:dynamicdata)
        n297 = call-poly <vilib>:"Mean.vi"("X"=w290) -> ("mean"=w292:dbl)  [unwired: 1 out]
        n298 = local read "editOffsetForce"() -> (w301:dbl)
        n299 = call "TCRef.vi"("offset"=w289, "data"=w303) -> ("emf(mV)"=w294:dbl, "temp (degC)"=w288:dbl)
        n300 = call-poly <vilib>:"Basic Level Trigger Detection.vi"("signal in"=w279, "level"=w273, "hysteresis"=w274, "error in (no error)"=w282) -> ("trigger detected?"=w278:bool, "error out"=w281:errorcluster)  [unwired: 9 in, 1 out]
        n301 = call "Thermocouple.vi"("cj(mV)"=w294, "factor"=301.8021, "data"=w292) -> ("temp(degC)"=w270:dbl)  [unwired: 2 out]
        n302 = call "LoadCell.vi"("tara"=w301, "factor"=w300, "data"=w295) -> ("force (Kgf)"=w297:dbl)
        n303 = local write "editTempRef"(w288) -> ()
        n304 = case shown="True" w278 {
          selector: w278 -> [w328 w329]
          tunnel: w261 -> [_ w330]
          tunnel: [_ w330] -> w280
          tunnel: [w328 w329] -> w277
          frame False {
          }
          frame True {
          }
        }
        "rpm" <- w277
        n305 = xnode ("Set Dynamic Data Attributes")("Signals In"=w323) -> ("Signals Out"=w309:dynamicdata, "error out"=w311:errorcluster)  [unwired: 4 in]
        n306 = local write "editForce"(w297) -> ()
        n307 = local read "ledBrake"() -> (w271:bool)
        n308 = xnode ("Set Dynamic Data Attributes")("Signals In"=w309, "error in"=w311) -> ("Signals Out"=w310:dynamicdata, "error out"=w312:errorcluster)  [unwired: 3 in]
        n309 = xnode ("Set Dynamic Data Attributes")("Signals In"=w310, "error in"=w312) -> ("Signals Out"=w324:dynamicdata, "error out"=w313:errorcluster)  [unwired: 3 in]
        n310 = call "Timing and Transition Measurements2"("error in (no error)"=w281, "Signals"=w280) -> ("error out"=→"error out":errorcluster, "Frequency"=w276:dynamicdata)  [unwired: 8 in]
        n311 = case shown="True" w271 {
          tunnel: w270 -> [_ w327]
          tunnel: [w326 w327] -> w269
          frame False {
            n312 = local read "editTempA"() -> (w326:dbl)
          }
          frame True {
          }
        }
        n313 = xnode ("Set Dynamic Data Attributes")("Signals In"=w324, "error in"=w313) -> ("Signals Out"=w325:dynamicdata, "error out"=w314:errorcluster)  [unwired: 3 in]
        n314 = To Double Precision Float(number=w276) -> (double precision float=w275:dbl)
        n315 = local read "Lower level"() -> (w272:dbl)
        n316 = local read "editSetSpeed"() -> (w296:dbl)
        n317 = xnode ("Set Dynamic Data Attributes")("Signals In"=w325, "error in"=w314) -> ("Signals Out"=w315:dynamicdata, "error out"=w316:errorcluster)  [unwired: 3 in]
        n318 = call "RPM.vi"("factor"=w296, "Lower level"=w272, "data"=w275) -> ("km/h"=w299:dbl, "RPM"=w298:dbl)  [unwired: 1 out]
        n319 = call "Write To Measurement File2"("Signals"=w315, "Enable"=w284, "error in (no error)"=w316, "Filename"=w308) -> ()  [unwired: 13 in, 3 out]
        n320 = local write "editEngineSpeed"(w298) -> ()
        n321 = local write "editSpeed"(w299) -> ()
        n322 = local write "editTempA"(w269) -> ()
        n323 = disable-structure shown="Enabled" {
          frame Enabled {
            n324 = property on="editSpeed" class="DigNum (strict)"() -> ("Value"=w331:dbl)  [unwired: 2 in, 2 out]
            n325 = property on="editSpeed" class="DigNum (strict)"("Val(Sgnl)"=w331) -> ()  [unwired: 2 in, 2 out]
          }
          frame Disabled {
            n326 = property on="velocidade 2" class="DigNum (strict)"() -> ("Value"=w332:u32)  [unwired: 2 in, 2 out]
            n327 = property on="velocidade" class="DigNum (strict)"("Val(Sgnl)"=w332) -> ()  [unwired: 2 in, 2 out]
          }
        }
      }
    }
    n328 = local read "buttonBrake"() -> (w257:bool)
    n329 = local read "buttonMotor"() -> (w255:bool)
    n330 = local read "ledBrake"() -> (w259:bool)
    n331 = local read "ledMotor"() -> (w256:bool)
    n332 = Or(x=w257, y=w259) -> (x .or. y?=w258:bool)
    n333 = Or(x=w255, y=w256) -> (x .or. y?=w254:bool)
    n334 = local read "deviceName"() -> (w248:tag)
    n335 = Build Array(w258, w254) -> (w260:bool[])
    n336 = call "DAQ Assistant2"("data"=w260, "stop (T)"=w253, "device name"=w248) -> ()  [unwired: 15 in, 2 out]
  }
  n337 = disable-structure shown="Disabled" {
    frame Disabled {
    }
    frame Enabled {
    }
  }
  "velocidade" <- "velocidade 2"
